vi "Network Steam Close.vi"(8 "error in (no error)":errorcluster, 11 "Model_AMC in":refnum<class "Model_AMC.lvclass">) -> (0 "error out":errorcluster, 3 "Model_AMC out":refnum<class "Model_AMC.lvclass">)   [LabVIEW 2021, in "Model_AMC.lvclass"]
uses:
  Model_AMC.lvclass
  Model_AMC.lvclass/Model_AMC.ctl
  <userlib>/John_Lib/Network_Streams_Connection/NetworkConnection.lvclass
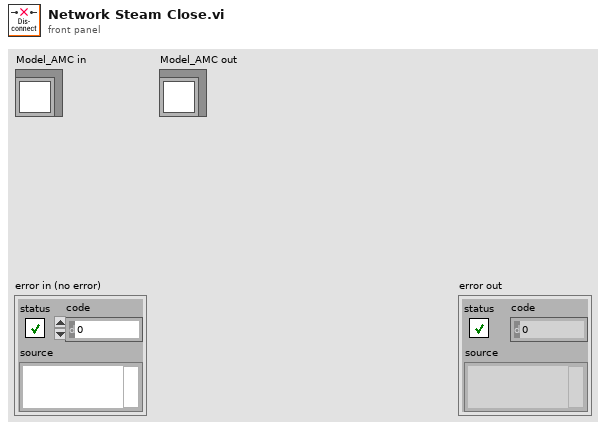
[diagram p1: front panel]
types:
  T1 = typedef "Model_AMC.lvclass/DVR.ctl" = cluster{"JKI_Network_Streams":refnum<class "NetworkConnection.lvclass">, "AMC Q":T2}
  T2 = typedef "Model_AMC.lvclass/AMC Q.ctl" = cluster{"Main":T3, "OPCUA":T3, "NetworkSteam":T3}
  T3 = typedef "AMC_FW.lvlib/Queue.ctl" = cluster{"Q":T4, "Name":string}
  T4 = typedef "AMC_FW.lvlib/Message Queue.ctl" = refnum<queue>
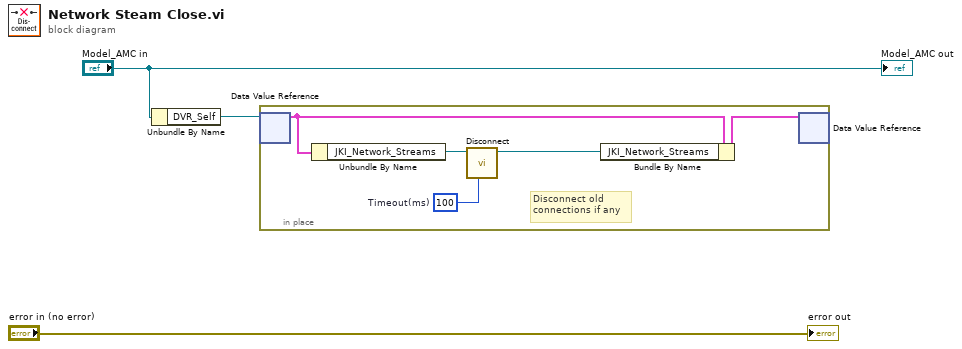
[diagram p0: block diagram]
diagram:
  n1 = Unbundle By Name("Model_AMC in") -> ("DVR_Self"=w2:refnum<data-value>)
  n2 = in-place {
    w8 = 100  # Timeout(ms)
    # "Disconnect old\nconnections if any"
    n3 = in-place-dvr #1(w2) -> (w7:T1)  [unwired: 1 out]
    n4 = Unbundle By Name(w7) -> ("JKI_Network_Streams"=w6:refnum<class "NetworkConnection.lvclass">)
    n5 = call <userlib>:"Disconnect.vi"("Timeout ms (1000)"=w8, "NetworkConnection in"=w6) -> ("NetworkConnection out"=w4:refnum<class "NetworkConnection.lvclass">)  [unwired: 8 in, 1 out]
    n6 = Bundle By Name(cluster=w7, "JKI_Network_Streams"=w4) -> (w5:T1)
    n7 = in-place-dvr #1(w5) -> ()  [unwired: 2 out]
  }
  "error out" <- "error in (no error)"
  "Model_AMC out" <- "Model_AMC in"
